vi "MyFIFOScheduler.vi"(8 "Processing Times (Rows Mach.Cols Jobs)":u16[][](array[numeric]), 9 "Number of Jobs":i32, 10 "Number of Machines":i32, 11 "Schedule":u16[](array[numeric])) -> (1 "Job Schedule on Machine":i32[][](array[numeric]), 3 "Gannt Chart Out":T1[][](array[typedef]))   [LabVIEW 2013, in "Scheduler.lvclass"]
uses:
  Scheduler.lvclass
  Controls/GanntChart_Element.ctl
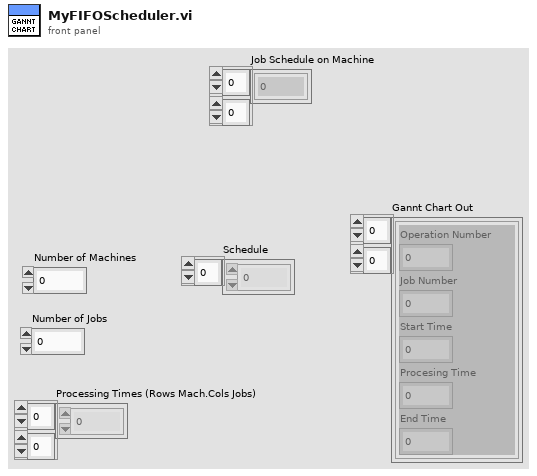
[diagram p1: front panel]
types:
  T1 = typedef "GanntChart_Element.ctl" = cluster{"Operation Number":i32, "Job Number":i32, "Start Time":i32, "Procesing Time":u16, "End Time":i32}
  T2 = typedef "Time_Interval_List_Element.ctl" = cluster{"Start Time":i32, "End Time":i32}
  T3 = typedef "Gap.ctl" = cluster{"Gap Start Time":i32, "Gap End Time":i32, "Gap Index":i32, "Operation Number":i32}
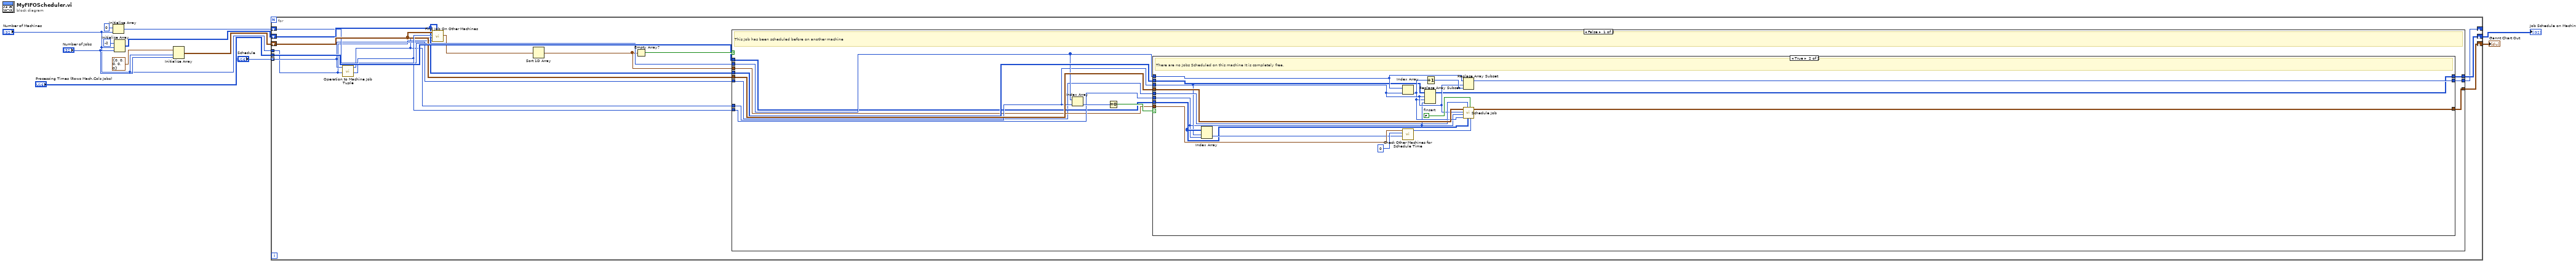
[diagram p0: block diagram]
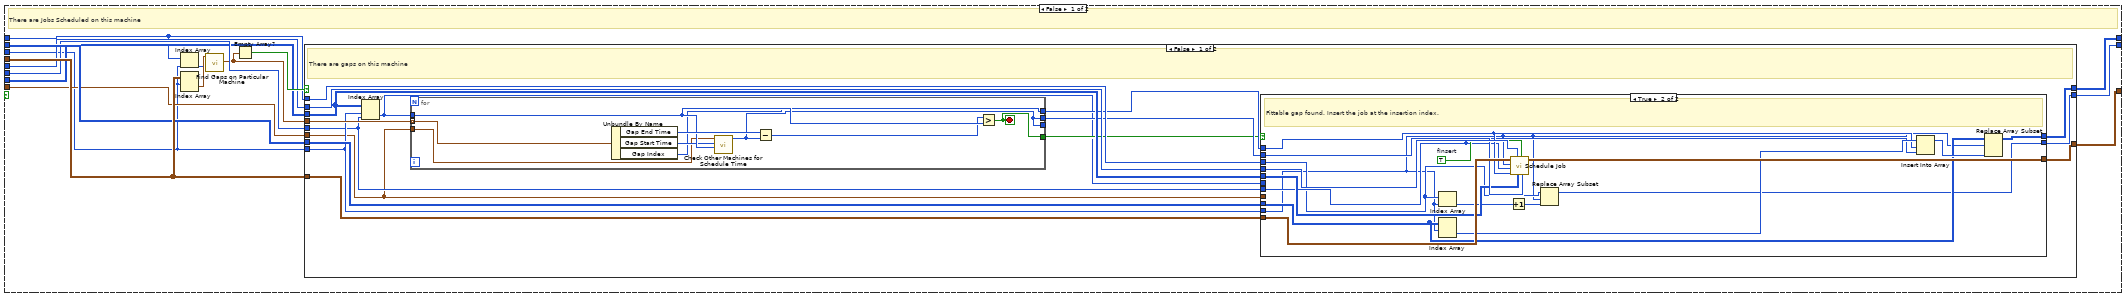
[diagram p2: hidden frame]
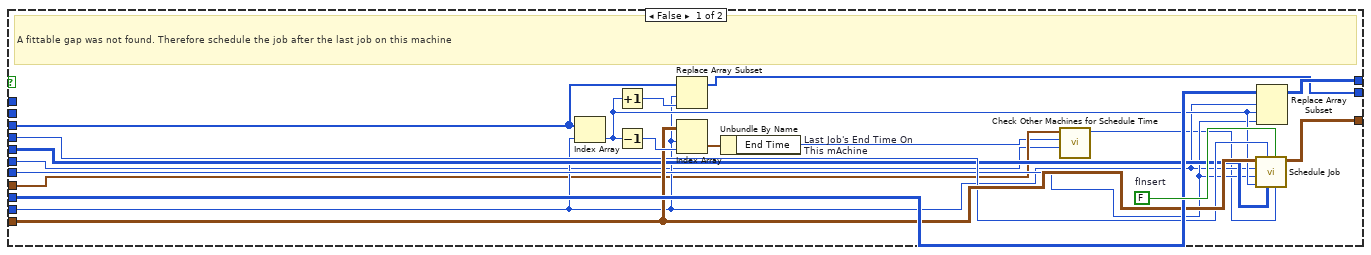
[diagram p3: hidden frame]
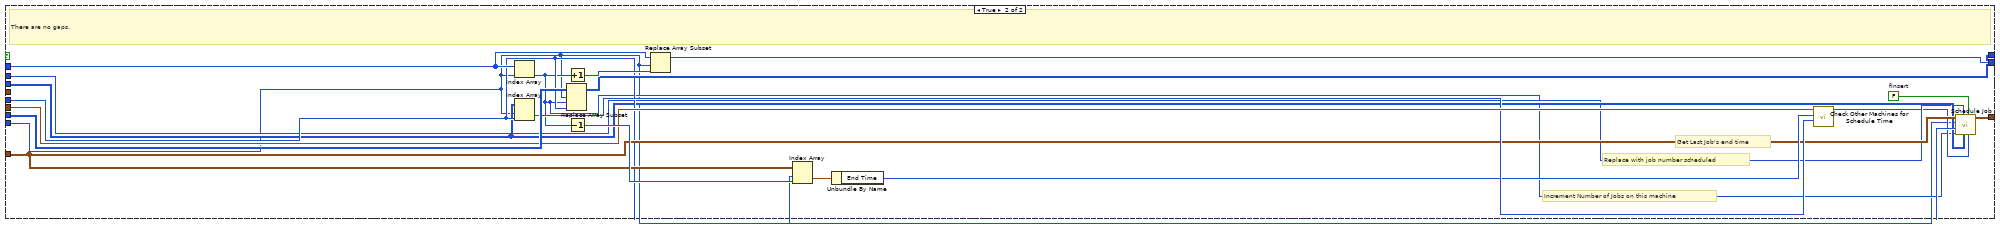
[diagram p4: hidden frame]
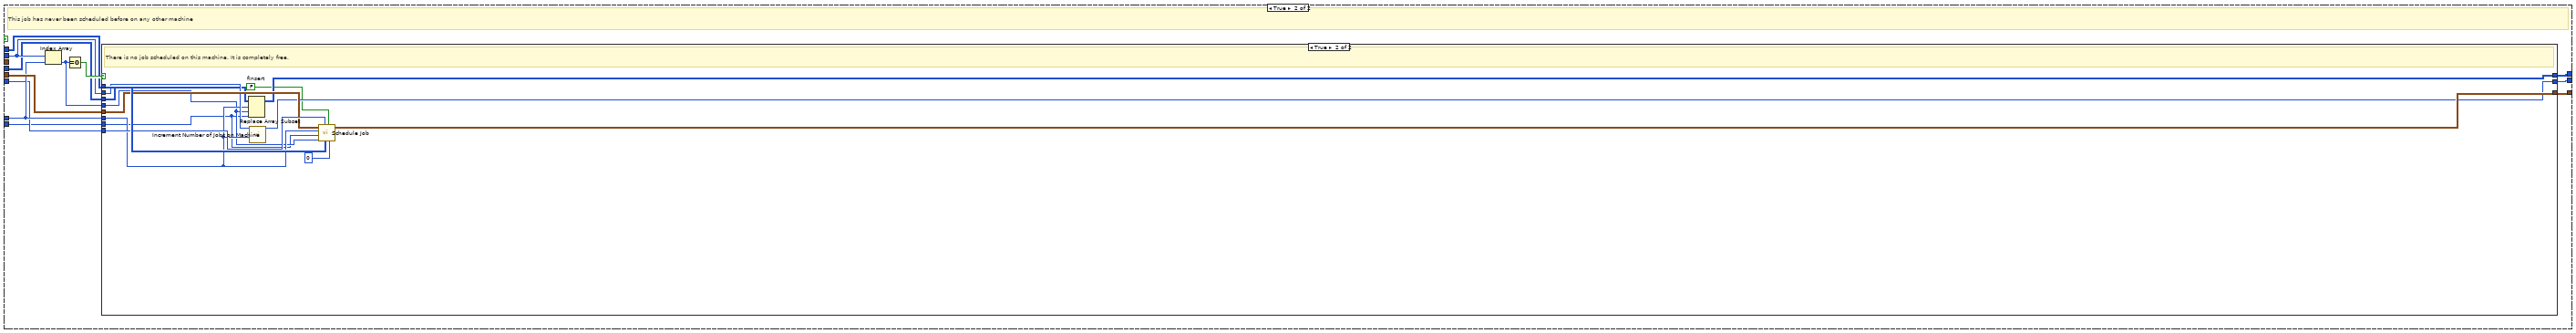
[diagram p5: hidden frame]
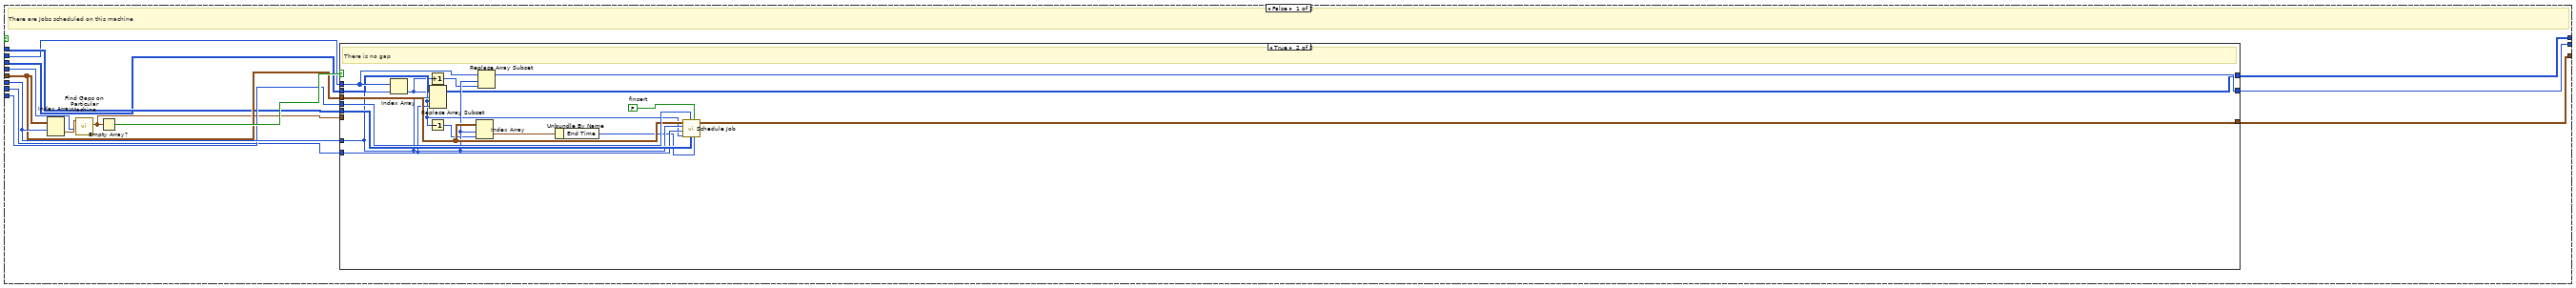
[diagram p6: hidden frame]
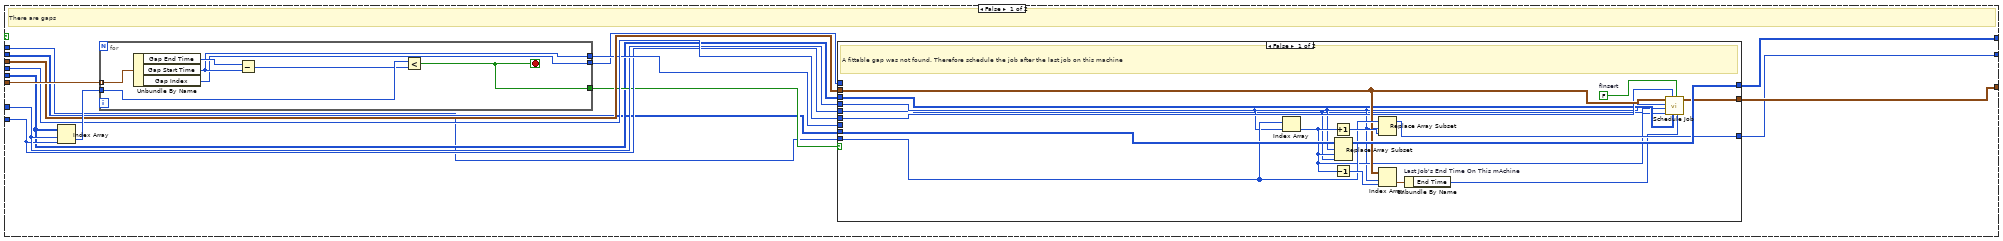
[diagram p7: hidden frame]
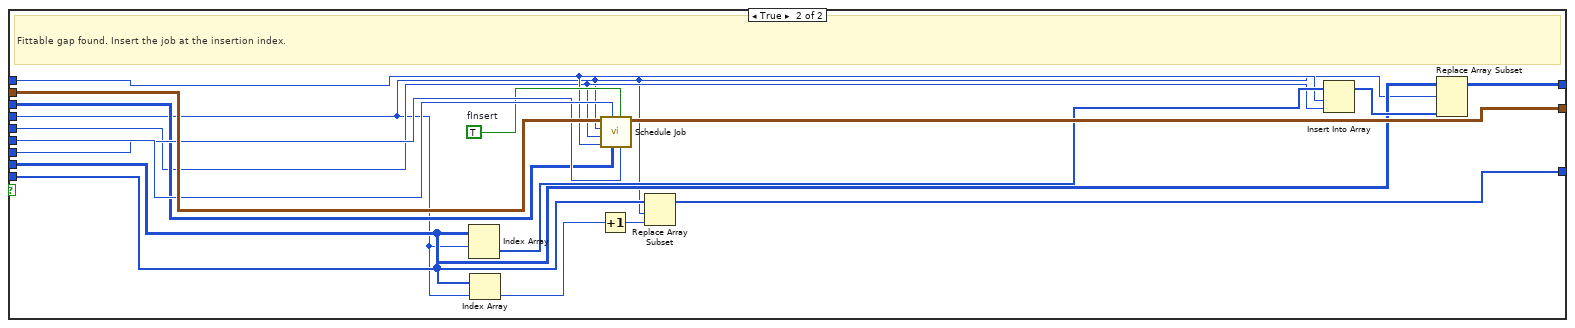
[diagram p8: hidden frame]
diagram:
  n1 = Initialize Array(0, "Number of Machines") -> (w4:i32[])
  n2 = Initialize Array(-2, "Number of Machines", "Number of Jobs") -> (w6:i32[][])
  n3 = Initialize Array(T1 {"Operation Number"=0, "Job Number"=0, "Start Time"=0, "Procesing Time"=0, "End Time"=0}, "Number of Machines", "Number of Jobs") -> (w2:T1[][])
  n4 = for {
    tunnel: "Schedule" -> [w19] mode=indexing
    tunnel: "Number of Machines" -> [w17]
    shift-right: [w13] -> w12
    shift-left: w2 -> [w23]
    tunnel: "Processing Times (Rows Mach.Cols Jobs)" -> [w25]
    shift-right: [w21] -> w1
    shift-left: w6 -> [w22]
    shift-right: [w18] -> _
    shift-left: w4 -> [w20]
    n5 = call "Operation to Machine Job Tuple.vi"("Number of Machines"=w17, "Operation Number"=w19) -> ("Job No"=w24:i32, "Machine No"=w14:i32)  [unwired: 8 in]
    n6 = call "Find Job On Other Machines.vi"("Job Schedule on Machines"=w22, "Number of Machines"=w17, "Machine No"=w14, "Job No"=w24, "Gannt Chart"=w23) -> ("Time Interval List"=w16:T2[])  [unwired: 6 in]
    n7 = Sort 1D Array(array=w16) -> (sorted array=w15:T2[])
    n8 = Empty Array?(array=w15) -> (empty?=w26:bool)
    n9 = case shown="False" w26 {
      tunnel: w25 -> [w28 w157]
      tunnel: w24 -> [w30 w158]
      tunnel: w23 -> [w38 w162]
      tunnel: [w37 w156] -> w13
      tunnel: w22 -> [w36 w153]
      tunnel: [w35 w152] -> w21
      tunnel: w14 -> [w31 w161]
      tunnel: w15 -> [w29 _]
      tunnel: w20 -> [w34 w155]
      tunnel: w19 -> [w27 w159]
      tunnel: [w33 w154] -> w18
      frame False {
        # "This Job has been scheduled before on another machine"
        n10 = Index Array(array=w34, index=w31) -> (element=w39:i32)
        n11 = Equal To 0?(x=w39) -> (x = 0?=w32:bool)
        n12 = case shown="True" w32 {
          tunnel: [w51 w147] -> w37
          tunnel: w38 -> [w52 w148]
          tunnel: w36 -> [w50 w136]
          tunnel: [w49 w135] -> w35
          tunnel: w34 -> [w43 w141]
          tunnel: [w48 w140] -> w33
          tunnel: w31 -> [w42 w139]
          tunnel: w30 -> [w47 w137]
          tunnel: w29 -> [w46 w151]
          tunnel: w28 -> [w45 w143]
          tunnel: w27 -> [w44 w145]
          frame False {
            # "There are Jobs Scheduled on this machine"
            n13 = Index Array(array=w43, index=w42) -> (element=w41:i32)
            n14 = Index Array(array=w52, index (row)=w42) -> (element=w54:T1[])  [unwired: 1 in]
            n15 = call "Find Gaps on Particular Machine.vi"("Number of Scheduled Jobs on This Machine"=w41, "Gannt Chart For Machine In"=w54) -> ("Gaps"=w40:T3[])  [unwired: 9 in]
            n16 = Empty Array?(array=w40) -> (empty?=w53:bool)
            n17 = case shown="False" w53 {
              tunnel: w52 -> [w65 w123]
              tunnel: [w64 w122] -> w51
              tunnel: [w66 w127] -> w49
              tunnel: w50 -> [w67 w128]
              tunnel: [w68 w129] -> w48
              tunnel: w43 -> [w69 w130]
              tunnel: w42 -> [w62 w116]
              tunnel: w47 -> [w60 w121]
              tunnel: w46 -> [w57 w126]
              tunnel: w45 -> [w61 w120]
              tunnel: w44 -> [w63 w119]
              tunnel: w40 -> [w70 _]
              frame False {
                # "There are gaps on this machine"
                n18 = Index Array(array=w61, index (row)=w62, index (col)=w60) -> (element=w55:u16)
                n19 = for {
                  tunnel: w70 -> [w110] mode=indexing
                  tunnel: w55 -> [w114]
                  tunnel: [w108] -> w59
                  tunnel: [w112] -> w58
                  tunnel: w57 -> [w111]
                  tunnel: [w108] -> _
                  tunnel: [w107] -> w56
                  stop <- w107 stop-if-true
                  n20 = Unbundle By Name(w110) -> ("Gap End Time"=w115:i32, "Gap Start Time"=w113:i32, "Gap Index"=w112:i32)
                  n21 = call "Check Other Machines for Schedule Time.vi"("Processing Time of the Job on This Machine"=w114, "Current Machine Available Time"=w113, "Time Interval List"=w111) -> ("Time to schedule"=w108:i32)  [unwired: 8 in]
                  n22 = Subtract(x=w115, y=w108) -> (x-y=w109:i32)
                  n23 = Greater?(x=w109, y=w114) -> (0:w107:bool)
                }
                n24 = case shown="True" w56 {
                  tunnel: w65 -> [w81 w106]
                  tunnel: [w80 w105] -> w64
                  tunnel: w63 -> [w79 w104]
                  tunnel: w59 -> [_ w103]
                  tunnel: w62 -> [w75 w92]
                  tunnel: w60 -> [w76 w98]
                  tunnel: w61 -> [w78 w102]
                  tunnel: w58 -> [_ w99]
                  tunnel: w67 -> [w87 w96]
                  tunnel: w69 -> [w83 w93]
                  tunnel: [w86 w95] -> w66
                  tunnel: [w82 w90] -> w68
                  tunnel: w57 -> [w74 _]
                  tunnel: w55 -> [w72 _]
                  frame False {
                    w88 = FALSE  # fInsert
                    # "A fittable gap was not found. Therefore schedule the job after the last job on this machine"
                    n25 = Index Array(array=w83, index=w75) -> (element=w77:i32)
                    n26 = Increment(x=w77) -> (x+1=w89:i32)
                    n27 = Decrement(x=w77) -> (x-1=w85:i32)
                    n28 = Replace Array Subset(array=w83, new element=w89, index=w75) -> (w82:i32[])
                    n29 = Index Array(array=w81, index (row)=w75, index (col)=w85) -> (element=w84:T1)
                    n30 = Unbundle By Name "Last Job's End Time On This mAchine"(w84) -> ("End Time"=w73:i32)
                    n31 = call "Check Other Machines for Schedule Time.vi"("Processing Time of the Job on This Machine"=w72, "Current Machine Available Time"=w73, "Time Interval List"=w74) -> ("Time to schedule"=w71:i32)  [unwired: 8 in]
                    n32 = call "Schedule Job.vi"("Start Time"=w71, "fInsert"=w88, "Processing Times"=w78, "Operation"=w79, "Index to schedule/Insert"=w77, "Job Number"=w76, "Machine No"=w75, "Gannt Chart In"=w81) -> ("Gannt Chart Out"=w80:T1[][])  [unwired: 3 in]
                    n33 = Replace Array Subset(array=w87, new element=w76, index (row)=w75, index (col)=w77) -> (w86:i32[][])
                  }
                  frame True {
                    w101 = TRUE  # fInsert
                    # "Fittable gap found. Insert the job at the insertion index."
                    n34 = Index Array(array=w96, index (row)=w92) -> (element=w100:i32[])  [unwired: 1 in]
                    n35 = Index Array(array=w93, index=w92) -> (element=w94:i32)
                    n36 = Increment(x=w94) -> (x+1=w91:i32)
                    n37 = call "Schedule Job.vi"("Start Time"=w103, "fInsert"=w101, "Processing Times"=w102, "Operation"=w104, "Index to schedule/Insert"=w99, "Job Number"=w98, "Machine No"=w92, "Gannt Chart In"=w106) -> ("Gannt Chart Out"=w105:T1[][])  [unwired: 3 in]
                    n38 = Replace Array Subset(array=w93, new element=w91, index=w92) -> (w90:i32[])
                    n39 = Insert Into Array(array=w100, index=w99, new element=w98) -> (w97:i32[])
                    n40 = Replace Array Subset(array=w96, new element=w97, index (row)=w92) -> (w95:i32[][])  [unwired: 1 in]
                  }
                }
              }
              frame True {
                w132 = FALSE  # fInsert
                # "Get Last Job's end time"
                # "Increment Number of Jobs on this machine"
                # "Replace with job number scheduled"
                # "There are no gaps."
                n41 = Index Array(array=w130, index=w116) -> (element=w117:i32)
                n42 = Index Array(array=w120, index (row)=w116, index (col)=w121) -> (element=w125:u16)
                n43 = Replace Array Subset(array=w128, new element=w121, index (row)=w116, index (col)=w117) -> (w127:i32[][])
                n44 = Increment(x=w117) -> (x+1=w133:i32)
                n45 = Decrement(x=w117) -> (x-1=w134:i32)
                n46 = Replace Array Subset(array=w130, new element=w133, index=w116) -> (w129:i32[])
                n47 = Index Array(array=w123, index (row)=w116, index (col)=w134) -> (element=w131:T1)
                n48 = Unbundle By Name(w131) -> ("End Time"=w124:i32)
                n49 = call "Check Other Machines for Schedule Time.vi"("Processing Time of the Job on This Machine"=w125, "Current Machine Available Time"=w124, "Time Interval List"=w126) -> ("Time to schedule"=w118:i32)  [unwired: 8 in]
                n50 = call "Schedule Job.vi"("Start Time"=w118, "fInsert"=w132, "Processing Times"=w120, "Operation"=w119, "Index to schedule/Insert"=w117, "Job Number"=w121, "Machine No"=w116, "Gannt Chart In"=w123) -> ("Gannt Chart Out"=w122:T1[][])  [unwired: 3 in]
              }
            }
          }
          frame True {
            w146 = FALSE  # fInsert
            # "There are no Jobs Scheduled on this machine It is completely free."
            n51 = Index Array(array=w143, index (row)=w139, index (col)=w137) -> (element=w149:u16)
            n52 = Index Array(array=w141, index=w139) -> (element=w138:i32)
            n53 = call "Check Other Machines for Schedule Time.vi"("Processing Time of the Job on This Machine"=w149, "Current Machine Available Time"=0, "Time Interval List"=w151) -> ("Time to schedule"=w144:i32)  [unwired: 8 in]
            n54 = Replace Array Subset(array=w136, new element=w137, index (row)=w139, index (col)=w138) -> (w135:i32[][])
            n55 = Increment(x=w138) -> (x+1=w142:i32)
            n56 = Replace Array Subset(array=w141, new element=w142, index=w139) -> (w140:i32[])
            n57 = call "Schedule Job.vi"("Start Time"=w144, "fInsert"=w146, "Processing Times"=w143, "Operation"=w145, "Index to schedule/Insert"=w138, "Job Number"=w137, "Machine No"=w139, "Gannt Chart In"=w148) -> ("Gannt Chart Out"=w147:T1[][])  [unwired: 3 in]
          }
        }
      }
      frame True {
        # "This job has never been scheduled before on any other machine"
        n58 = Index Array(array=w155, index=w161) -> (element=w160:i32)
        n59 = Equal To 0?(x=w160) -> (x = 0?=w163:bool)
        n60 = case shown="True" w163 {
          tunnel: w162 -> [w174 w258]
          tunnel: w161 -> [w175 w254]
          tunnel: w160 -> [w164 w253]
          tunnel: w159 -> [w172 w259]
          tunnel: w158 -> [w171 w252]
          tunnel: w157 -> [w170 w261]
          tunnel: [w173 w260] -> w156
          tunnel: [w167 w256] -> w154
          tunnel: w155 -> [w168 w257]
          tunnel: w153 -> [w166 w255]
          tunnel: [w165 w251] -> w152
          frame False {
            # "There are Jobs scheduled on this machine"
            n61 = Index Array(array=w174, index (row)=w175) -> (element=w177:T1[])  [unwired: 1 in]
            n62 = call "Find Gaps on Particular Machine.vi"("Number of Scheduled Jobs on This Machine"=w164, "Gannt Chart For Machine In"=w177) -> ("Gaps"=w169:T3[])  [unwired: 9 in]
            n63 = Empty Array?(array=w169) -> (empty?=w176:bool)
            n64 = case shown="True" w176 {
              tunnel: w174 -> [w190 w246]
              tunnel: w168 -> [w179 w244]
              tunnel: w175 -> [w186 w241]
              tunnel: [w189 w248] -> w173
              tunnel: w172 -> [w188 w247]
              tunnel: w171 -> [w185 w240]
              tunnel: w170 -> [w183 w245]
              tunnel: w169 -> [w192 _]
              tunnel: [w178 w243] -> w167
              tunnel: w166 -> [w181 w242]
              tunnel: [w180 w239] -> w165
              frame False {
                # "There are gaps"
                n65 = Index Array(array=w183, index (row)=w186, index (col)=w185) -> (element=w191:u16)
                n66 = for {
                  tunnel: w192 -> [w232] mode=indexing
                  tunnel: w191 -> [w230]
                  tunnel: [w228] -> w187
                  tunnel: [w227] -> w184
                  tunnel: [w226] -> w182
                  stop <- w227 stop-if-true
                  n67 = Unbundle By Name(w232) -> ("Gap End Time"=w231:i32, "Gap Start Time"=w228:i32, "Gap Index"=w226:i32)
                  n68 = Subtract(x=w231, y=w228) -> (x-y=w229:i32)
                  n69 = Less?(x=w230, y=w229) -> (x < y?=w227:bool)
                }
                n70 = case shown="False" w184 {
                  tunnel: w190 -> [w199 w225]
                  tunnel: [w198 w224] -> w189
                  tunnel: w188 -> [w197 w223]
                  tunnel: w187 -> [_ w222]
                  tunnel: w186 -> [w194 w211]
                  tunnel: w185 -> [w193 w217]
                  tunnel: w183 -> [w196 w221]
                  tunnel: w182 -> [_ w218]
                  tunnel: w181 -> [w206 w215]
                  tunnel: w179 -> [w202 w212]
                  tunnel: [w205 w214] -> w180
                  tunnel: [w201 w209] -> w178
                  frame False {
                    w207 = FALSE  # fInsert
                    # "A fittable gap was not found. Therefore schedule the job after the last job on this machine"
                    n71 = Index Array(array=w202, index=w194) -> (element=w195:i32)
                    n72 = Increment(x=w195) -> (x+1=w208:i32)
                    n73 = Decrement(x=w195) -> (x-1=w204:i32)
                    n74 = Replace Array Subset(array=w206, new element=w193, index (row)=w194, index (col)=w195) -> (w205:i32[][])
                    n75 = Replace Array Subset(array=w202, new element=w208, index=w194) -> (w201:i32[])
                    n76 = Index Array(array=w199, index (row)=w194, index (col)=w204) -> (element=w203:T1)
                    n77 = Unbundle By Name "Last Job's End Time On This mAchine"(w203) -> ("End Time"=w200:i32)
                    n78 = call "Schedule Job.vi"("Start Time"=w200, "fInsert"=w207, "Processing Times"=w196, "Operation"=w197, "Index to schedule/Insert"=w195, "Job Number"=w193, "Machine No"=w194, "Gannt Chart In"=w199) -> ("Gannt Chart Out"=w198:T1[][])  [unwired: 3 in]
                  }
                  frame True {
                    w220 = TRUE  # fInsert
                    # "Fittable gap found. Insert the job at the insertion index."
                    n79 = Index Array(array=w215, index (row)=w211) -> (element=w219:i32[])  [unwired: 1 in]
                    n80 = Index Array(array=w212, index=w211) -> (element=w213:i32)
                    n81 = Increment(x=w213) -> (x+1=w210:i32)
                    n82 = call "Schedule Job.vi"("Start Time"=w222, "fInsert"=w220, "Processing Times"=w221, "Operation"=w223, "Index to schedule/Insert"=w218, "Job Number"=w217, "Machine No"=w211, "Gannt Chart In"=w225) -> ("Gannt Chart Out"=w224:T1[][])  [unwired: 3 in]
                    n83 = Replace Array Subset(array=w212, new element=w210, index=w211) -> (w209:i32[])
                    n84 = Insert Into Array(array=w219, index=w218, new element=w217) -> (w216:i32[])
                    n85 = Replace Array Subset(array=w215, new element=w216, index (row)=w211) -> (w214:i32[][])  [unwired: 1 in]
                  }
                }
              }
              frame True {
                w233 = FALSE  # fInsert
                # "There is no gap"
                n86 = Index Array(array=w244, index=w241) -> (element=w234:i32)
                n87 = Increment(x=w234) -> (x+1=w235:i32)
                n88 = Decrement(x=w234) -> (x-1=w238:i32)
                n89 = Replace Array Subset(array=w242, new element=w240, index (row)=w241, index (col)=w234) -> (w239:i32[][])
                n90 = Index Array(array=w246, index (row)=w241, index (col)=w238) -> (element=w237:T1)
                n91 = Replace Array Subset(array=w244, new element=w235, index=w241) -> (w243:i32[])
                n92 = Unbundle By Name(w237) -> ("End Time"=w236:i32)
                n93 = call "Schedule Job.vi"("Start Time"=w236, "fInsert"=w233, "Processing Times"=w245, "Operation"=w247, "Index to schedule/Insert"=w234, "Job Number"=w240, "Machine No"=w241, "Gannt Chart In"=w246) -> ("Gannt Chart Out"=w248:T1[][])  [unwired: 3 in]
              }
            }
          }
          frame True {
            w249 = FALSE  # fInsert
            # "There is no job scheduled on this machine. It is completely free."
            n94 = Replace Array Subset(array=w255, new element=w252, index (row)=w254, index (col)=w253) -> (w251:i32[][])
            n95 = call "Increment Number of Jobs on Machine.vi"("Machine Number"=w254, "Number of Jobs Scheduled On Machines in"=w257) -> ("Number of Jobs Scheduled On Machines out"=w256:i32[])  [unwired: 9 in]
            n96 = call "Schedule Job.vi"("Start Time"=0, "fInsert"=w249, "Processing Times"=w261, "Operation"=w259, "Index to schedule/Insert"=w253, "Job Number"=w252, "Machine No"=w254, "Gannt Chart In"=w258) -> ("Gannt Chart Out"=w260:T1[][])  [unwired: 3 in]
          }
        }
      }
    }
  }
  "Gannt Chart Out" <- w12
  "Job Schedule on Machine" <- w1
